vi "data_input.vi"() -> ()   [LabVIEW 2026]
uses:
  <vilib>/DAQmx/read.llb/DAQmx Read.vi
  <vilib>/DAQmx/read.llb/DAQmx Read (Analog 1D Wfm NChan NSamp).vi
  <vilib>/DAQmx/miscellaneous.llb/DAQmx Fill In Error Info.vi
panel:
  out "data":waveform(dbl)[](graph)
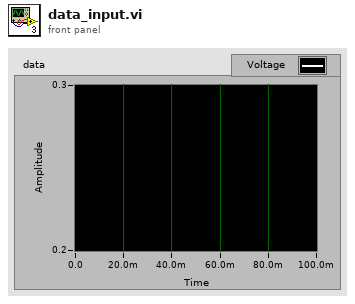
[diagram p1: front panel]
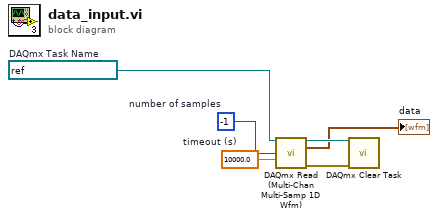
[diagram p0: block diagram]
diagram:
  w5 = 10000.0  # timeout (s)
  w6 = -1  # number of samples
  w2 = refnum<k21> "MyVoltageTask"  # DAQmx Task Name
  n1 = call-poly "DAQmx Read (Multi-Chan Multi-Samp 1D Wfm).vi"("task/channels in"=w2, "number of samples per channel"=w6, "timeout"=w5) -> ("task out"=w3:refnum<k21>, "data"=→"data":waveform(dbl)[], "error out"=w4:errorcluster)  [unwired: 10 in]
  n2 = call <vilib>:"DAQmx Clear Task.vi"("task in"=w3, "error in"=w4) -> ()  [unwired: 13 in, 1 out]
